vi "Initialize Hardware References.vi"(8 "error in (no error)":errorcluster, 11 "Hardware Resources in":T1={"DAQmx Channel"="", "Sample Rate"=0.0, "DAQmx Task"="", "ResetInterp"=FALSE, "GainConstants"=[2.0, 10.0, 1.0, 0.1, 0.01, 0.001], "FilterCoefficients"=[], "ChannelNames"=[], "ActiveChannels"=[], "Display Rate"=1000, "ResponseExtension"=TRUE}) -> (0 "error out":errorcluster, 3 "Hardware Resources out":T1={"DAQmx Channel"="", "Sample Rate"=0.0, "DAQmx Task"="", "ResetInterp"=FALSE, "GainConstants"=[2.0, 10.0, 1.0, 0.1, 0.01, 0.001], "FilterCoefficients"=[], "ChannelNames"=[], "ActiveChannels"=[], "Display Rate"=1000, "ResponseExtension"=TRUE})   [LabVIEW 2017, in "Acquisition.lvlib"]
doc: "Initialize the hardware references."
uses:
  Acquisition.lvlib
  Hardware Configuration.ctl
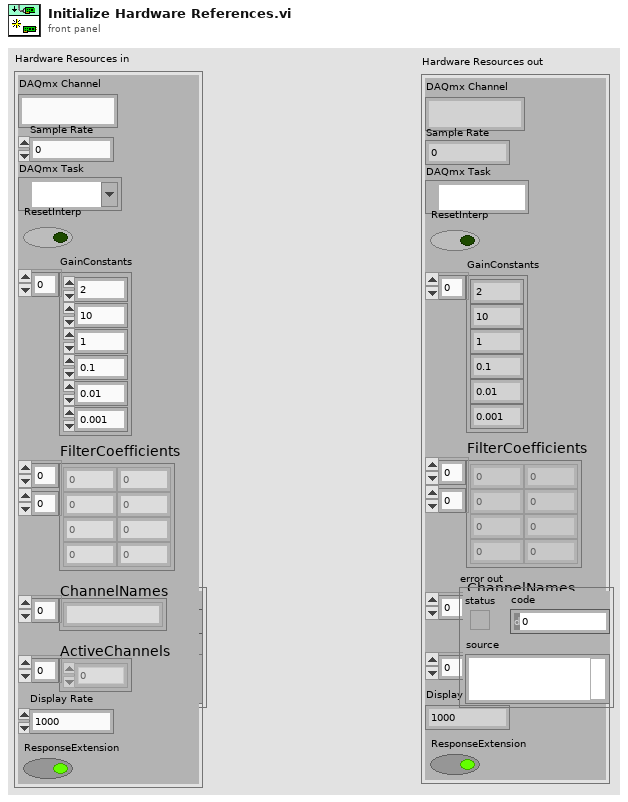
[diagram p1: front panel]
types:
  T1 = typedef "Acquisition.lvlib/Hardware Configuration.ctl" = cluster{"DAQmx Channel":string, "Sample Rate":dbl, "DAQmx Task":refnum<k21>, "ResetInterp":bool, "GainConstants":dbl[], "FilterCoefficients":dbl[][], "ChannelNames":string[], "ActiveChannels":i32[], "Display Rate":i32, "ResponseExtension":bool}
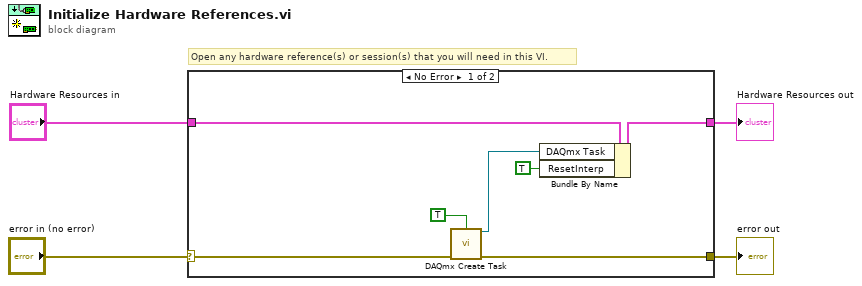
[diagram p0: block diagram]
diagram:
  # "Open any hardware reference(s) or session(s) that you will need in this VI."
  n1 = case shown="No Error" "error in (no error)" {
    selector: "error in (no error)" -> [w8 w12]
    tunnel: [w6 w12] -> w3
    tunnel: "Hardware Resources in" -> [w10 w13]
    tunnel: [w11 w13] -> w1
    frame No Error {
      n2 = call <vilib>:"DAQmx Create Task.vi"("auto cleanup"=TRUE, "error in"=w8) -> ("task out"=w7:refnum<k21>, "error out"=w6:errorcluster)  [unwired: 12 in]
      n3 = Bundle By Name(cluster=w10, "DAQmx Task"=w7, "ResetInterp"=TRUE) -> (w11:T1)
    }
    frame Error {
    }
  }
  "Hardware Resources out" <- w1
  "error out" <- w3
